vi "Analyze Temperature (broken Run button).vi"() -> ()   [LabVIEW 2020]
uses:
  <vilib>/DAQmx/read.llb/DAQmx Read (Analog DBL 1Chan 1Samp).vi
  <vilib>/DAQmx/create/channels.llb/DAQmx Create Channel (AI-Temperature-Thermocouple).vi
  <vilib>/DAQmx/miscellaneous.llb/DAQmx Fill In Error Info.vi
panel:
  out "In Range ?":bool
  out "Current Temperature (deg F)":dbl
  out "Current Temperature (deg C)":dbl
  in  "Lower Limit (deg C)":dbl
  in  "Upper Limit (deg C)":dbl
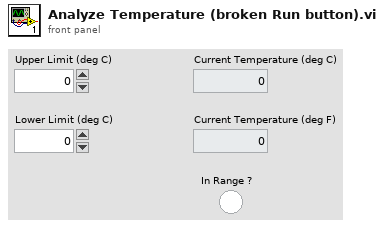
[diagram p1: front panel]
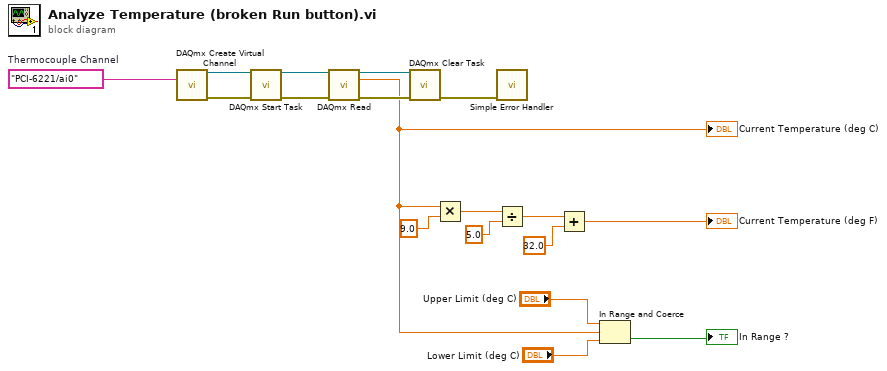
[diagram p0: block diagram]
diagram:
  w18 = tag "PCI-6221/ai0"  # Thermocouple Channel
  n1 = call-poly <vilib>:"DAQmx Create Virtual Channel.vi"("physical channels"=w18) -> ("task out"=w17:refnum<k21>, "error out"=w16:errorcluster)  [unwired: 13 in]
  n2 = call <vilib>:"DAQmx Start Task.vi"("task/channels in"=w17, "error in"=w16) -> ("task out"=w15:refnum<k21>, "error out"=w14:errorcluster)  [unwired: 12 in]
  n3 = call-poly <vilib>:"DAQmx Read.vi"("task/channels in"=w15, "error in"=w14) -> ("task out"=w13:refnum<k21>, "data"=w4:dbl, "error out"=w12:errorcluster)  [unwired: 11 in]
  "Current Temperature (deg C)" <- w4
  n4 = call <vilib>:"DAQmx Clear Task.vi"("task in"=w13, "error in"=w12) -> ("error out"=w1:errorcluster)  [unwired: 13 in]
  n5 = Multiply(x=w4, y=9.0) -> (x*y=w10:dbl)
  n6 = call <vilib>:"Simple Error Handler.vi"("error in (no error)"=w1) -> ()  [unwired: 4 in, 5 out]
  n7 = Divide(x=w10, y=5.0) -> (x/y=w9:dbl)
  n8 = Add(x=w9, y=32.0) -> (x+y=→"Current Temperature (deg F)":dbl)
  n9 = In Range and Coerce(upper limit="Upper Limit (deg C)", x=w4, lower limit="Lower Limit (deg C)") -> (In Range?=→"In Range ?":bool)  [unwired: 1 out]
